vi "NIMS_DF_iir_comb(n, bw, ab, t).vi"(7 "type":enum32{"notch", "peak"}(ring), 9 "ab":dbl=3.010299956639812 format="%#.6g", 10 "bw":dbl=0.02 format="%.2f", 11 "n":i32) -> (0 "error":i32, 2 "a":dbl[](array[numeric]), 3 "b":dbl[](array[numeric]))   [LabVIEW 2017, in "NI_DigFilter_MathScript.lvlib"]
uses:
  <vilib>/addons/Digital Filter Design/NI_DigFilter_MathScript.lvlib
  <vilib>/addons/Digital Filter Design/Design.llb/DFD IIR Comb Design by N and BW.vi
  <vilib>/addons/Digital Filter Design/NI_DigFilterLicensed.lvlib
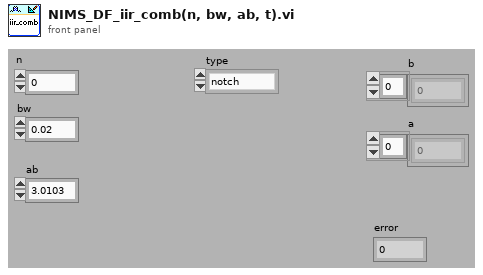
[diagram p1: front panel]
types:
  T1 = enum16{"Notch Type I", "Notch Type II", "Peak Type I", "Peak Type II"}
  T2 = typedef "NI_DigFilterLicensed.lvlib/DFD Filter Obj.ctl" = cluster{"mSRate_Fs":dbl, "mSRate_Version":string, "mSRate_Comments":string, "mSRate_OrgCoef":T3, "mSRate_CurCoef":T3, "mSRate_Quantized?":bool, "mSRate_QCoef":T3, "mSRate_QSettings":T5[], "mSRate_Order":i32, "mSRate_Scaling":cluster{"mSRate_ScaleByPowerOf2?":bool, "mSRate_ScaleType":T7}}
  T3 = typedef "NI_DigFilterLicensed.lvlib/DFD Filter Coef.ctl" = cluster{"type":T4, "gain":dbl, "coef a (k)":dbl[], "coef b (v)":dbl[]}
  T4 = typedef "NI_DigFilterLicensed.lvlib/DFD Filter Structure Type Selector.ctl" = enum16{"Undefined", "FIR Direct Form", "FIR Direct Form Transposed", "FIR Symmetric", "FIR Antisymmetric", "IIR Direct Form I", "IIR Direct Form I Transposed", "IIR Direct Form II", "IIR Direct Form II Transposed", "IIR Cascaded Second Order Sections Form I", "IIR Cascaded Second Order Sections Form I Transposed", "IIR Cascaded Second Order Sections Form II", "IIR Cascaded Second Order Sections Form II Transposed", "Lattice Allpass (basic sections)", "Lattice Allpass (one multiplier sections)", "Lattice Allpass (normalized sections)", "Lattice AR (basic sections)", "Lattice AR (one multiplier sections)", "Lattice AR (normalized sections)", "Lattice MA (minimum phase)", "Lattice MA (maximum phase)", "Lattice ARMA (basic sections)", "Lattice ARMA (one multiplier sections)", "Lattice ARMA (normalized sections)"}
  T5 = typedef "NI_DigFilterLicensed.lvlib/dfd_Internal Quantization Settings.ctl" = cluster{"source":T6, "wl":i16, "iwl":i16, "overflow mode":enum16{"Saturation", "Wrap"}, "rounding mode":enum16{"Nearest", "Truncation"}, "signed?":bool}
  T6 = typedef "NI_DigFilterLicensed.lvlib/dfd_Internal Quantization Srcs.ctl" = u16
  T7 = typedef "NI_DigFilterLicensed.lvlib/DFD Coef Norm Type.ctl" = enum16{"No Norm", "Time Domain 1-Norm", "Time Domain 2-Norm", "Time Domain Inf-Norm"}
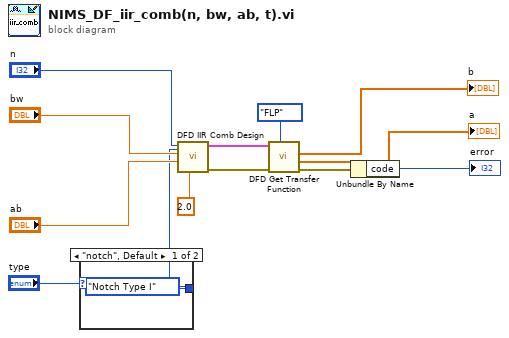
[diagram p0: block diagram]
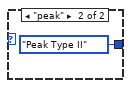
[diagram p2: hidden frame]
diagram:
  n1 = case shown="\"notch\", Default" "type" {
    tunnel: [T1."Notch Type I" ("filter type") T1."Peak Type II" ("filter type")] -> w3
    frame "notch", Default {
    }
    frame "peak" {
    }
  }
  n2 = call-poly <vilib>:"DFD IIR Comb Design.vi"("fs [Hz]"=2.0, "filter type"=w3, "Ab [dB]"="ab", "Df [Hz]"="bw", "# notches/peaks"="n") -> ("error out"=w8:errorcluster, "filter out"=w9:T2)  [unwired: 1 in, 4 out]
  n3 = call <vilib>:"DFD Get Transfer Function.vi"("type (FLP)"=enum16{"FLP", "FXP"}."FLP", "error in (no error)"=w8, "filter in"=w9) -> ("error out"=w12:errorcluster, "denominator"=→"a":dbl[], "numerator"=→"b":dbl[])  [unwired: 6 out]
  n4 = Unbundle By Name(w12) -> ("code"=→"error":i32)
